vi "testSensor.vi"() -> ()   [LabVIEW 2018]
uses:
  Sensor/SensorShared/clSensorData.ctl
  Sensor/SensorPlugins/PmuBaseClass/Typedef/PmuData.ctl
  Sensor/SensorModule/SensorModule.lvlib
  Sensor/SensorShared/SensorShared.lvlib
  Sensor/SensorPlugins/PmuBaseClass/PmuBase.lvclass
panel:
  out "time stamp":timestamp
  out "Numeric":u64
  in  "stop":bool
  out "ModuleID":i32
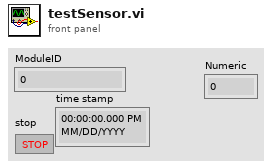
[diagram p1: front panel]
types:
  T1 = typedef "SensorShared.lvlib/clBroadcastEvents.ctl" = cluster{"DidInit":refnum<user-event>, "StatusUpdate":refnum<user-event>, "ErrorReport":refnum<user-event>, "DidStop":refnum<user-event>, "PathToINI":refnum<user-event>, "SensorReport":refnum<user-event>, "SensorConfig":refnum<user-event>}
  T2 = typedef "SensorPlugins.lvlib/PmuBase.lvclass/PmuData.ctl" = cluster{"Timestamp":dbl, "Synx":cdb[], "Freq":dbl, "ROCOF":dbl, "ID":i16}
  T3 = typedef "SensorShared.lvlib/clSensorData.ctl" = cluster{"SensorType":string, "SensorData":variant}
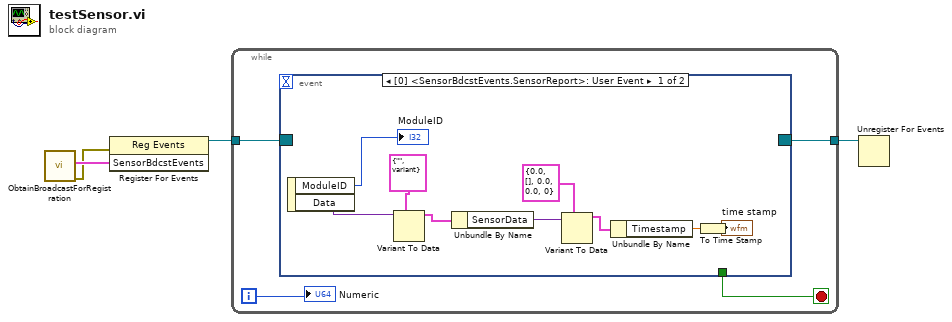
[diagram p0: block diagram]
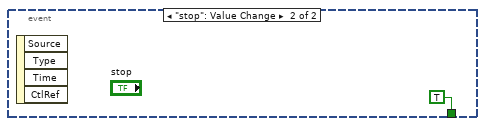
[diagram p2: hidden frame]
diagram:
  n1 = call "ObtainBroadcastForRegistration.vi"() -> ("error out"=w3:errorcluster, "SensorBdcstEvents"=w4:T1)  [unwired: 10 in]
  n2 = register-events(error in=w3, w4) -> (reference out=w2:refnum<event-registration>)  [unwired: 1 in, 1 out]
  n3 = while {
    tunnel: w2 -> [w8]
    tunnel: [w7] -> w1
    i -> [w5]
    stop <- w6 stop-if-true
    n4 = event shown="[0] <SensorBdcstEvents.SensorReport>: User Event" {
      selector: w8 -> [_ _]
      dyn-events: [_ _] -> w7
      timeout: _ -> [_ _]
      tunnel: [_ TRUE] -> w6
      event User Event {
        n5 = event-data() -> ("ModuleID"=→"ModuleID":i32, "Data"=w17:variant)  [unwired: 1 in]
        n6 = Variant To Data(type=T3 {"SensorType"="", "SensorData"=variant} ("clSensorData"), Variant=w17) -> (data=w15:T3)  [unwired: 1 in, 1 out]
        n7 = Unbundle By Name(w15) -> ("SensorData"=w14:variant)
        n8 = Variant To Data(type=T2 {"Timestamp"=0.0, "Synx"=[], "Freq"=0.0, "ROCOF"=0.0, "ID"=0} ("PmuReport"), Variant=w14) -> (data=w12:T2)  [unwired: 1 in, 1 out]
        n9 = Unbundle By Name(w12) -> ("Timestamp"=w11:dbl)
        n10 = To Time Stamp(1:w11) -> (0:→"time stamp":timestamp)
      }
      event "stop": Value Change {
        n11 = event-data() -> ()  [unwired: 1 in, 4 out]
      }
    }
    "Numeric" <- w5
  }
  n12 = Unregister For Events(event registration refnum=w1) -> ()  [unwired: 1 in, 1 out]
